vi "straight.vi"() -> ()   [LabVIEW 2009]
uses:
  <vilib>/Analysis/NI_AALBase.lvlib
panel:
  in  "増幅率":dbl
  out "歪み率(%)":dbl
  in  "ホワイトノイズの最大振幅":dbl
  out "DC":cluster{dbl[], dbl[]}(graph)
  out "AC":cluster{dbl[], dbl[]}(graph)
  in  "カットオフ周波数(Hz)":dbl
  in  "Q":dbl
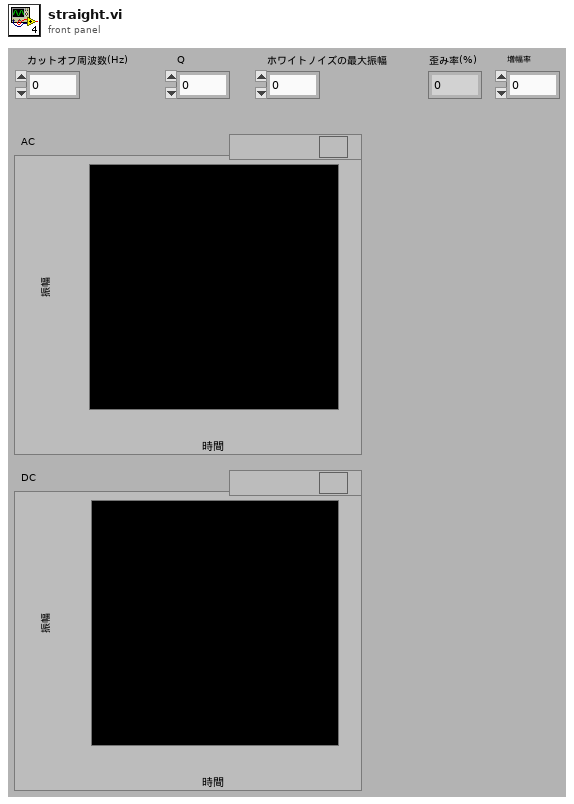
[diagram p1: front panel]
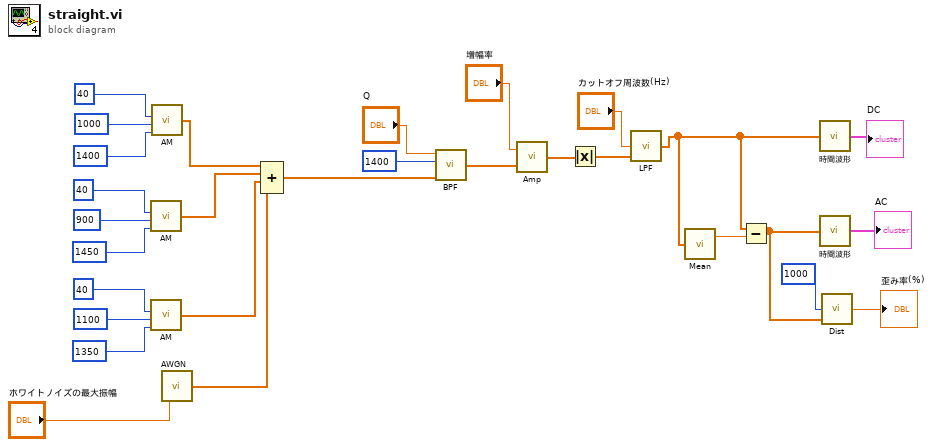
[diagram p0: block diagram]
diagram:
  n1 = call "AM.vi"("変調度 [%]"=40, "変調周波数 [Hz]"=900, "搬送波周波数 [kHz]"=1450) -> ("変調波"=w19:dbl[])  [unwired: 2 in]
  n2 = call "AM.vi"("変調度 [%]"=40, "変調周波数 [Hz]"=1100, "搬送波周波数 [kHz]"=1350) -> ("変調波"=w18:dbl[])  [unwired: 2 in]
  n3 = call "AM.vi"("変調度 [%]"=40, "変調周波数 [Hz]"=1000, "搬送波周波数 [kHz]"=1400) -> ("変調波"=w20:dbl[])  [unwired: 2 in]
  n4 = call "AWGN.vi"("振幅値"="ホワイトノイズの最大振幅") -> ("出力"=w17:dbl[])
  n5 = Compound Arithmetic op=ADD(w20, w19, w18, w17) -> (w16:dbl[])
  n6 = call "BPF.vi"("X"=w16, "中心周波数 [kHz]"=1400, "Q"="Q") -> ("BPF出力"=w14:dbl[])  [unwired: 1 in]
  n7 = call "Amp.vi"("入力"=w14, "増幅率"="増幅率") -> ("出力"=w12:dbl[])
  n8 = Absolute Value(x=w12) -> (abs(x)=w11:dbl[])
  n9 = call "LPF.vi"("入力"=w11, "カットオフ周波数 [Hz]"="カットオフ周波数(Hz)") -> ("LPF出力"=w8:dbl[])  [unwired: 1 in]
  n10 = call <vilib>:"Mean.vi"("X"=w8) -> ("mean"=w9:dbl)  [unwired: 1 out]
  n11 = Subtract(x=w8, y=w9) -> (x-y=w3:dbl[])
  n12 = call "時間波形.vi"("入力"=w8) -> ("時間波形"=→"DC":cluster{dbl[], dbl[]})
  n13 = call "時間波形.vi"("入力"=w3) -> ("時間波形"=→"AC":cluster{dbl[], dbl[]})
  n14 = call "Dist.vi"("入力"=w3, "基本周波数 [Hz]"=1000) -> ("ひずみ率"=→"歪み率(%)":dbl)  [unwired: 1 in]
